vi "机械手顺序状态机.vi"(8 "error in (no error)":errorcluster caption="错误输入（无错误）", 11 "Start":bool) -> (0 "error out":errorcluster caption="错误输出", 3 "Data Out":T1)   [LabVIEW 2013]
uses:
  Control/Data.ctl
  Control/YV.ctl
  Control/SW.ctl
  Control/State.ctl
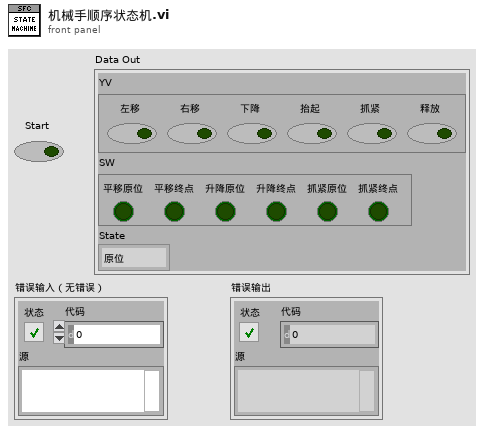
[diagram p1: front panel]
types:
  T1 = typedef "Data.ctl" = cluster{"YV":T2, "SW":T3, "State":T4}
  T2 = typedef "YV.ctl" = cluster{"左移":bool, "右移":bool, "下降":bool, "抬起":bool, "抓紧":bool, "释放":bool}
  T3 = typedef "SW.ctl" = cluster{"平移原位":bool, "平移终点":bool, "升降原位":bool, "升降终点":bool, "抓紧原位":bool, "抓紧终点":bool}
  T4 = typedef "State.ctl" = enum16{"原位", "A侧下降", "夹紧工件", "A侧抬起", "右移", "B侧下降", "释放工件", "B侧抬起", "左移"}
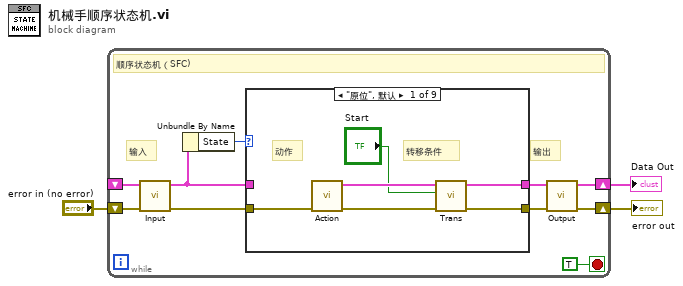
[diagram p0: block diagram]
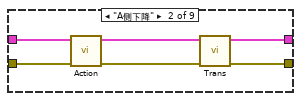
[diagram p2: hidden frame]
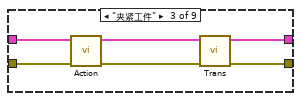
[diagram p3: hidden frame]
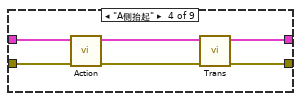
[diagram p4: hidden frame]
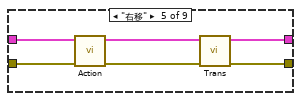
[diagram p5: hidden frame]
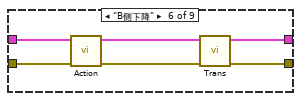
[diagram p6: hidden frame]
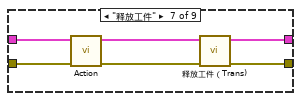
[diagram p7: hidden frame]
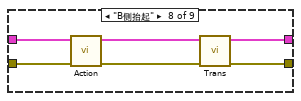
[diagram p8: hidden frame]
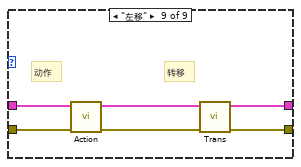
[diagram p9: hidden frame]
diagram:
  n1 = while {
    shift-right: [w9] -> w1
    shift-left: _ -> [w7]
    shift-right: [w8] -> w2
    shift-left: "error in (no error)" -> [w6]
    stop <- TRUE stop-if-true
    # "输出"
    # "输入"
    # "顺序状态机（SFC)"
    n2 = call "Input.vi"("error in (no error)"=w6, "Data In"=w7) -> ("error out"=w5:errorcluster, "Data Out"=w4:T1)  [unwired: 8 in]
    n3 = Unbundle By Name(w4) -> ("State"=w12:T4)
    n4 = case shown="\"原位\", 默认" w12 {
      tunnel: w5 -> [w19 w25 w31 w37 w43 w49 w55 w61 w67]
      tunnel: [w15 w22 w28 w34 w40 w46 w52 w58 w64] -> w11
      tunnel: [w14 w21 w27 w33 w39 w45 w51 w57 w63] -> w10
      tunnel: w4 -> [_ w20 w26 w32 w38 w44 w50 w56 w62]
      frame "原位", Default {
        # "转移条件"
        # "动作"
        n5 = call-poly "Action.vi"("error in (no error)"=w19) -> ("error out"=w17:errorcluster, "Data Out"=w18:T1)  [unwired: 9 in]
        n6 = call-poly "Trans.vi"("error in (no error)"=w17, "Start"="Start", "Data In"=w18) -> ("error out"=w14:errorcluster, "Data Out"=w15:T1)  [unwired: 7 in]
      }
      frame "A侧下降" {
        n7 = call-poly "Action.vi"("error in (no error)"=w25, "Data In"=w20) -> ("error out"=w24:errorcluster, "Data Out"=w23:T1)  [unwired: 8 in]
        n8 = call-poly "Trans.vi"("error in (no error)"=w24, "Data In"=w23) -> ("error out"=w21:errorcluster, "Data Out"=w22:T1)  [unwired: 8 in]
      }
      frame "夹紧工件" {
        n9 = call-poly "Action.vi"("error in (no error)"=w31, "Data In"=w26) -> ("error out"=w29:errorcluster, "Data Out"=w30:T1)  [unwired: 8 in]
        n10 = call-poly "Trans.vi"("error in (no error)"=w29, "Data In"=w30) -> ("error out"=w27:errorcluster, "Data Out"=w28:T1)  [unwired: 8 in]
      }
      frame "A侧抬起" {
        n11 = call-poly "Action.vi"("error in (no error)"=w37, "Data In"=w32) -> ("error out"=w35:errorcluster, "Data Out"=w36:T1)  [unwired: 8 in]
        n12 = call-poly "Trans.vi"("error in (no error)"=w35, "Data In"=w36) -> ("error out"=w33:errorcluster, "Data Out"=w34:T1)  [unwired: 8 in]
      }
      frame "右移" {
        n13 = call-poly "Action.vi"("error in (no error)"=w43, "Data In"=w38) -> ("error out"=w42:errorcluster, "Data Out"=w41:T1)  [unwired: 8 in]
        n14 = call-poly "Trans.vi"("error in (no error)"=w42, "Data In"=w41) -> ("error out"=w39:errorcluster, "Data Out"=w40:T1)  [unwired: 8 in]
      }
      frame "B侧下降" {
        n15 = call-poly "Action.vi"("error in (no error)"=w49, "Data In"=w44) -> ("error out"=w47:errorcluster, "Data Out"=w48:T1)  [unwired: 8 in]
        n16 = call-poly "Trans.vi"("error in (no error)"=w47, "Data In"=w48) -> ("error out"=w45:errorcluster, "Data Out"=w46:T1)  [unwired: 8 in]
      }
      frame "释放工件" {
        n17 = call-poly "Action.vi"("error in (no error)"=w55, "Data In"=w50) -> ("error out"=w54:errorcluster, "Data Out"=w53:T1)  [unwired: 8 in]
        n18 = call "释放工件（Trans).vi"("error in (no error)"=w54, "Data In"=w53) -> ("error out"=w51:errorcluster, "Data Out"=w52:T1)  [unwired: 8 in]
      }
      frame "B侧抬起" {
        n19 = call-poly "Action.vi"("error in (no error)"=w61, "Data In"=w56) -> ("error out"=w59:errorcluster, "Data Out"=w60:T1)  [unwired: 8 in]
        n20 = call-poly "Trans.vi"("error in (no error)"=w59, "Data In"=w60) -> ("error out"=w57:errorcluster, "Data Out"=w58:T1)  [unwired: 8 in]
      }
      frame "左移" {
        # "转移"
        # "动作"
        n21 = call-poly "Action.vi"("error in (no error)"=w67, "Data In"=w62) -> ("error out"=w65:errorcluster, "Data Out"=w66:T1)  [unwired: 8 in]
        n22 = call-poly "Trans.vi"("error in (no error)"=w65, "Data In"=w66) -> ("error out"=w63:errorcluster, "Data Out"=w64:T1)  [unwired: 8 in]
      }
    }
    n23 = call "Output.vi"("error in (no error)"=w10, "Data In"=w11) -> ("error out"=w8:errorcluster, "Data Out"=w9:T1)  [unwired: 8 in]
  }
  "error out" <- w2
  "Data Out" <- w1
